vi "Fast SQL Query v1_0_0.vi"(7 "Transpose?":bool=TRUE, 8 "error in (no error)":errorcluster, 10 "SQL":string="EXEC GET_BUTTON_BY_PERMISSION 1,2", 11 "connection reference":T1=refnum) -> (0 "error out":errorcluster, 1 "1D Data out":string[](array[string])=["Test Reports\t2\t\t\t0\t-1\t\t0\t\t\t"], 2 "2D Data out":string[][](table)=[["Test Reports"], ["2"], [""], [""], ["0"], ["-1"], [""], ["0"], [""], [""], [""]], 3 "dup connection reference":T1, 5 "Single Out":string="Test Reports\t2\t\t\t0\t-1\t\t0\t\t\t\r")   [LabVIEW 2009]
doc: "Fast SQL Query v1_0_0.vi\n\nVI is used to search databases through the ActiveX control Module. this Vi searches the entire database at one time. This is a much more effecient search than that used by the NI Database Connectivity Toolset.\n\nCreated 2002\nby National Analytics\nJ.Daren Suntych and Jim Teresigni"
uses:
  <vilib>/addons/database/Connection.llb/Conn ObjectReference.ctl
  <vilib>/addons/database/Recordset.llb/Rec Destroy - Connection.vi
  <vilib>/addons/database/Connection.llb/Conn Execute.vi
  <vilib>/addons/database/NI_Database_API.lvlib
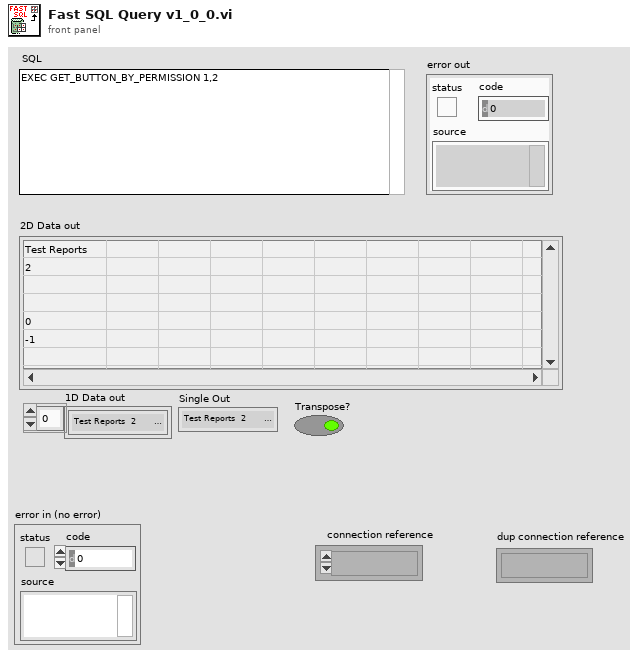
[diagram p1: front panel]
types:
  T1 = typedef "NI_Database_API.lvlib/Conn ObjectReference.ctl" = refnum<k1>
  T2 = typedef "NI_Database_API.lvlib/Rec ObjectReference.ctl" = refnum<k1>
  T3 = typedef "NI_Database_API.lvlib/Rec DataMembers.ctl" = cluster{"ADODB._Recordset":refnum<k7>, "Connection":T1}
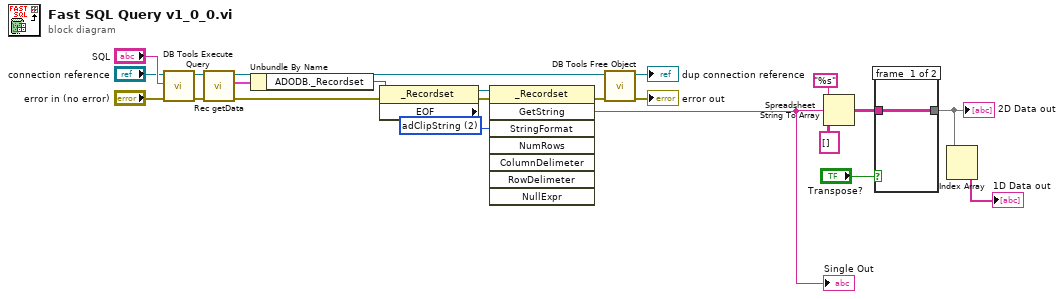
[diagram p0: block diagram]
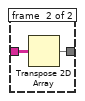
[diagram p2: hidden frame]
diagram:
  w1 = 2 items=["adClipString"=2] ("StringFormat")
  n1 = call-poly <vilib>:"DB Tools Execute Query.vi"("error in (no error)"="error in (no error)", "SQL query"="SQL", "connection reference"="connection reference") -> ("error out"=w20:errorcluster, "recordset reference"=w12:T2)  [unwired: 1 in, 4 out]
  n2 = call <vilib>:"Rec getData.vi"("error in (no error)"=w20, "recordset reference"=w12) -> ("error out"=w9:errorcluster, "data"=w21:T3, "recordset reference out"=w19:T2)  [unwired: 3 out]
  n3 = Unbundle By Name(w21) -> ("ADODB._Recordset"=w8:refnum<k7>)
  n4 = property class="_Recordset" props=["EOF"](reference=w8, error in=w9) -> (reference out=w7:refnum<k7>, error out=w10:errorcluster)  [unwired: 1 out]
  n5 = invoke class="_Recordset" method="GetString"(reference=w7, error in=w10, "StringFormat"=w1) -> (error out=w6:errorcluster, "GetString"=w5:string)  [unwired: 5 in, 6 out]
  "Single Out" <- w5
  n6 = call-poly <vilib>:"DB Tools Free Object.vi"("error in (no error)"=w6, "recordset reference"=w19) -> ("error out"=→"error out":errorcluster, "connection reference"=→"dup connection reference":T1)  [unwired: 8 out]
  n7 = Spreadsheet String To Array(format string="%s", spreadsheet string=w5, array type (2D Dbl)=string[][] []) -> (array=w16:string[][])  [unwired: 1 out]
  n8 = case shown="True" "Transpose?" {
    tunnel: w16 -> [w23 w25]
    tunnel: [w23 w24] -> w4
    frame #0 {
    }
    frame #1 {
      n9 = Transpose 2D Array(2D array=w25) -> (transposed array=w24:string[][])
    }
  }
  "2D Data out" <- w4
  n10 = Index Array(array=w4) -> (element=→"1D Data out":string[])  [unwired: 2 in]
